vi "Zad3.vi"() -> ()   [LabVIEW 2015]
panel:
  in  "OldVal 2":string
  out "NewVal":string
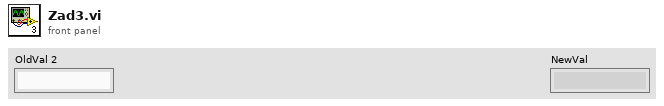
[diagram p1: front panel]
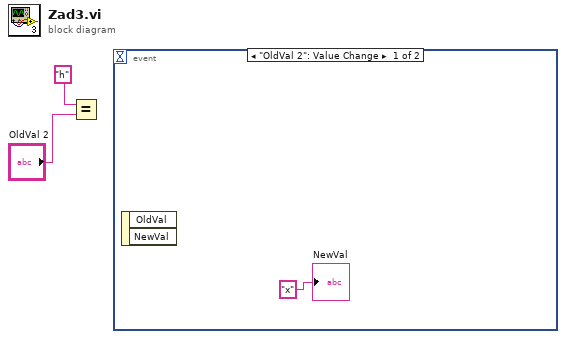
[diagram p0: block diagram]
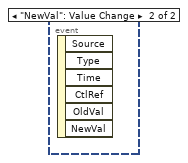
[diagram p2: hidden frame]
diagram:
  n1 = Equal?(x="h", y="OldVal 2") -> ()  [unwired: 1 out]
  n2 = event shown="[0] \"OldVal 2\": Value Change" {
    selector: _ -> [_ _]
    dyn-events: _ -> [_ _]
    timeout: _ -> [_ _]
    event "OldVal 2": Value Change {
      n3 = event-data() -> ()  [unwired: 1 in, 2 out]
      "NewVal" <- "x"
    }
    event "NewVal": Value Change {
      n4 = event-data() -> ()  [unwired: 1 in, 6 out]
    }
  }
